vi "Read Requirements Filepath.vi"(11 "Project in":refnum<class "RequirementsMap.lvclass">) -> (2 "File Path":path, 3 "Project out":refnum<class "RequirementsMap.lvclass">)   [LabVIEW 2021, in "Bananas.lvlib" / "RequirementsMap.lvclass"]
uses:
  RequirementsMap.lvclass
  RequirementsMap.lvclass/RequirementsMap.ctl
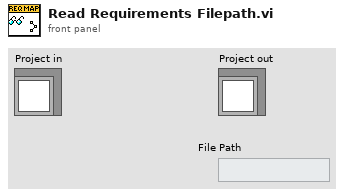
[diagram p1: front panel]
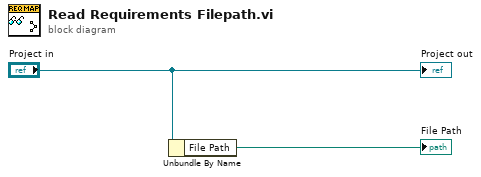
[diagram p0: block diagram]
diagram:
  n1 = Unbundle By Name("Project in") -> ("File Path"=→"File Path":path)
  "Project out" <- "Project in"
